vi "SeCrTs-Datalog Redundant .vi"() -> ()   [LabVIEW 2022 SP3]
uses:
  Source Code/Globals/SeCrTs-RD globals.vi
  0df20dd4-2c00-4f15-959c-8f534c1a7d29.vi
  97d5b880-568e-4530-a46e-1f8a36fc1bc1.vi
panel:
  in  "EXIT":bool
  out "log heath":bool
  out "Connected?":bool
  in  "Ip address":string="169.254.92.239"
  out "error out":errorcluster
  in  "error in":errorcluster
  # "DATALOG REDUNDANT V1.0"
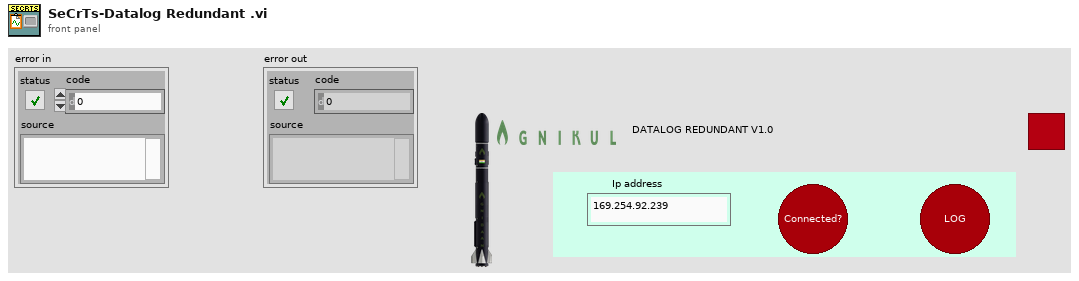
[diagram p1: front panel]
types:
  T1 = cluster{"AO config":cluster{"Channel_Name":string, "Channel_Number":string, "Default_Value":dbl, "Units":string}[], "AI config":cluster{"Channel_Name":string, "Channel_Number":string, "Pre_Scale_min":dbl, "Pre_Scale_max":dbl, "Sensor_min":dbl, "Sensor_max":dbl, "Units":string}[], "DI config":cluster{"Channel_Name":string, "Channel_Number":string, "Default_Value":bool, "DI invert?":bool}[], "DO config":cluster{"Channel_Name":string, "Channel_Number":string, "Default_Value":bool, "DO invert?":bool}[], "TC config":cluster{"Channel_Name":string, "Channel_Number":string, "Pre_Scale_min":dbl, "Pre_Scale_max":dbl, "units":i32, " type":i32}[], "ACC config":cluster{"Channel_Name":string, "Channel_Number":string, "Pre_Scale_min":dbl, "Pre_Scale_max":dbl, "Terminal configuration":i32, "Sensitivity":dbl, "Sensitivity units":i32}[], "SG config":cluster{"Channel_Name":string, "Channel_Number":string, "Pre_Scale_min":dbl, "Pre_Scale_max":dbl}[], "Strain Gauge Settings":cluster{"poisson ratio":dbl, "nominal gage resistance":dbl, "gage factor":dbl}, "Bridge Settings":cluster{"voltage excitation value":dbl, "voltage excitation source":i32, "initial bridge voltage":dbl, "lead wire resistance":dbl, "strain configuration":i32}, "Sample Rate":cluster{"AI Sample Rate":dbl[], "AO Sample Rate":dbl[], "DI Sample Rate":dbl[], "TC Sample Rate":dbl[], "DO Sample Rate":dbl[], "SG Sample Rate":dbl[], "ACC Sample Rate":dbl[]}}
  T2 = cluster{"analog names":cluster{"AI_C_Data":string[], "AI_V_Data":string[], "AO_Data":string[], "DO_Data":string[], "ACC_Data":string[], "TC Data":string[], "Drive_A_C":string[], "Drive_A_D":string[], "Drive_L_C":string[], "Drive_L_D":string[]}, "Di names":string[]}
  T3 = cluster{"AI_C_Data":string[], "AI_V_Data":string[], "AO_Data":string[], "DO_Data":string[], "ACC_Data":string[], "TC Data":string[], "Drive_A_C":string[], "Drive_A_D":string[], "Drive_L_C":string[], "Drive_L_D":string[]}
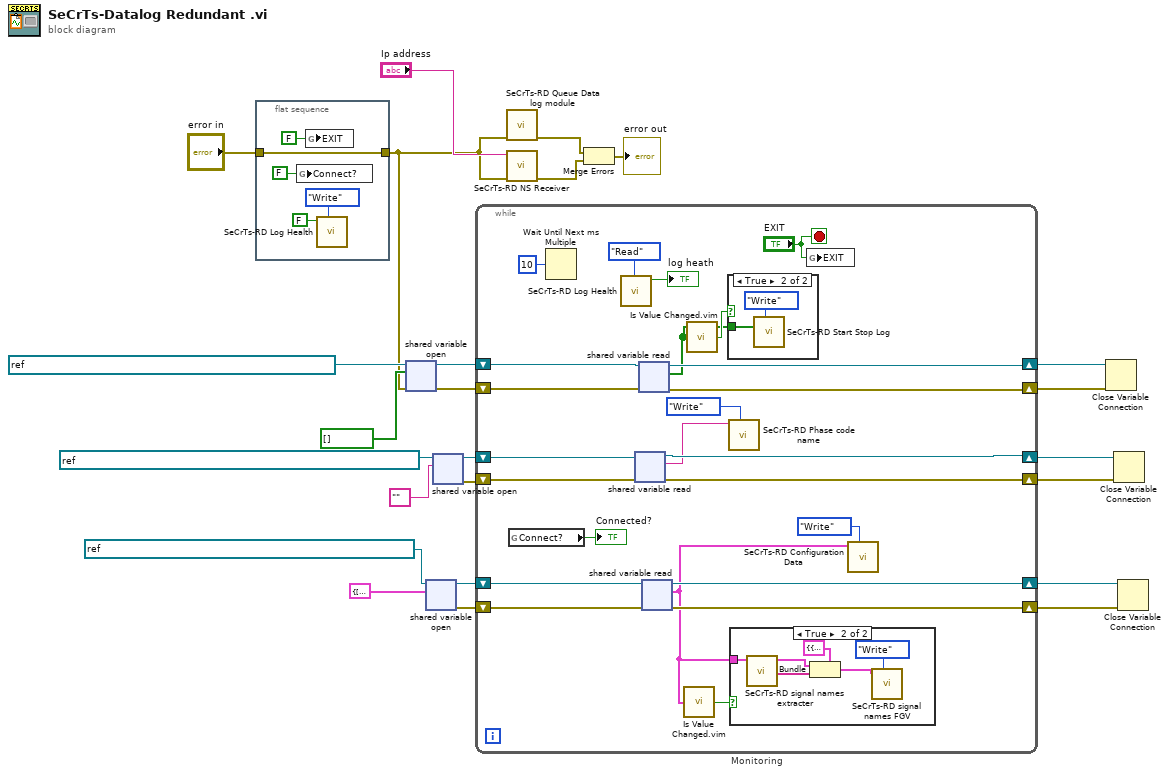
[diagram p0: block diagram]
diagram:
  n1 = flat-sequence {
    tunnel: "error in" -> [w28]
    tunnel: [w28] -> w14
    frame #0 {
      n2 = global write "SeCrTs-RD globals.vi" "Connect?"(FALSE ("Connect?")) -> ()
      n3 = global write "SeCrTs-RD globals.vi" "EXIT"(FALSE ("EXIT")) -> ()
      n4 = call "SeCrTs-RD Log Health.vi"("Enum"=enum16{"Read", "Write"}."Write", "Log health"=FALSE) -> ()  [unwired: 8 in, 2 out]
    }
  }
  n5 = shared-variable-open(refnum<k21> "ni.var.psp://ni-pxie-8861-0326ae8e/Device/Start Stop log" ("shared variable refnum in"), w14, bool[] []) -> (w16:refnum<k21>, w15:errorcluster)  [unwired: 1 in]
  n6 = shared-variable-open(refnum<k21> "ni.var.psp://ni-pxie-8861-0326ae8e/Device/Configuration" ("shared variable refnum in"), T1 {"AO config"=[], "AI config"=[], "DI config"=[], "DO config"=[], "TC config"=[], "ACC config"=[], "SG config"=[], "Strain Gauge Settings"={"poisson ratio"=0.3, "nominal gage resistance"=120.0, "gage factor"=2.08}, "Bridge Settings"={"voltage excitation value"=3.3, "voltage excitation source"=10200, "initial bridge voltage"=0.0, "lead wire resistance"=1.7, "strain configuration"=10271}, "Sample Rate"={"AI Sample Rate"=[], "AO Sample Rate"=[], "DI Sample Rate"=[], "TC Sample Rate"=[], "DO Sample Rate"=[], "SG Sample Rate"=[], "ACC Sample Rate"=[]}} ("data")) -> (w6:refnum<k21>, w4:errorcluster)  [unwired: 2 in]
  n7 = shared-variable-open(refnum<k21> "ni.var.psp://ni-pxie-8861-0326ae8e/Device/Datalog phase code" ("shared variable refnum in"), "") -> (w10:refnum<k21>, w9:errorcluster)  [unwired: 2 in]
  n8 = while "Monitoring" {
    shift-right: [w47] -> w13
    shift-left: w16 -> [w48]
    shift-right: [w45] -> w12
    shift-left: w15 -> [w46]
    shift-right: [w42] -> w7
    shift-left: w10 -> [w44]
    shift-right: [w41] -> w8
    shift-left: w9 -> [w43]
    shift-right: [w33] -> w2
    shift-left: w6 -> [w36]
    shift-right: [w32] -> w1
    shift-left: w4 -> [w35]
    stop <- "EXIT" stop-if-true
    n9 = global read "SeCrTs-RD globals.vi" "Connect?"() -> (→"Connected?":bool)
    n10 = Wait Until Next ms Multiple(millisecond multiple=u32 10) -> ()  [unwired: 1 out]
    n11 = call "SeCrTs-RD Log Health.vi"("Enum"=enum16{"Read", "Write"}."Read") -> ("Log health R"=→"log heath":bool)  [unwired: 9 in, 1 out]
    n12 = shared-variable-read(w44, w43) -> (w42:refnum<k21>, w41:errorcluster, w39:string)  [unwired: 1 out]
    n13 = shared-variable-read(w48, w46) -> (w47:refnum<k21>, w45:errorcluster, w37:bool[])  [unwired: 1 out]
    n14 = shared-variable-read(w36, w35) -> (w33:refnum<k21>, w32:errorcluster, w31:T1)  [unwired: 1 out]
    n15 = call "Is Value Changed.vim"("value"=w31) -> ("changed or first call?"=w30:bool)
    n16 = call "Is Value Changed.vim"("value"=w37) -> ("changed or first call?"=w38:bool)
    n17 = case shown="True" w38 {
      tunnel: w37 -> [_ w60]
      frame False {
      }
      frame True {
        n18 = call "SeCrTs-RD Start Stop Log.vi"("Enum"=enum16{"Read", "Write"}."Write", "Start Stop log"=w60) -> ()  [unwired: 8 in, 2 out]
      }
    }
    n19 = call "SeCrTs-RD Phase code name.vi"("Enum"=enum16{"Read", "Write"}."Write", "Phase code W"=w39) -> ()  [unwired: 8 in, 2 out]
    n20 = case shown="True" w30 {
      tunnel: w31 -> [_ w59]
      frame False {
      }
      frame True {
        n21 = call "SeCrTs-RD signal names extracter.vi"("input cluster"=w59) -> ("Di names"=w56:string[], "analog names"=w57:T3)  [unwired: 9 in]
        n22 = Bundle(cluster=T2 {"analog names"={"AI_C_Data"=[], "AI_V_Data"=[], "AO_Data"=[], "DO_Data"=[], "ACC_Data"=[], "TC Data"=[], "Drive_A_C"=[], "Drive_A_D"=[], "Drive_L_C"=[], "Drive_L_D"=[]}, "Di names"=[]}, "analog names"=w57, "Di names"=w56) -> (w55:T2)
        n23 = call "SeCrTs-RD signal names FGV.vi"("Enum"=enum16{"Read", "Write"}."Write", "Signal names"=w55) -> ()  [unwired: 8 in, 2 out]
      }
    }
    n24 = global write "SeCrTs-RD globals.vi" "EXIT"("EXIT") -> ()
    n25 = call "SeCrTs-RD Configuration Data.vi"("Enum"=enum16{"Read", "Write"}."Write", "data"=w31) -> ()  [unwired: 8 in, 2 out]
  }
  n26 = call "SeCrTs-RD Queue Data log module.vi"("error in"=w14) -> ("error out"=w24:errorcluster)  [unwired: 10 in]
  n27 = call "SeCrTs-RD NS Receiver.vi"("error in"=w14, 11:"Ip address") -> ("error out"=w23:errorcluster)  [unwired: 9 in]
  n28 = Merge Errors(w24, w23) -> (→"error out":errorcluster)
  n29 = Close Variable Connection(8:w12, 11:w13) -> ()  [unwired: 1 out]
  n30 = Close Variable Connection(8:w8, 11:w7) -> ()  [unwired: 1 out]
  n31 = Close Variable Connection(8:w1, 11:w2) -> ()  [unwired: 1 out]
